vi "String Join.vi"(2 "separator (\\t)":string, 3 "string array":string[](array[string])) -> (0 "joined string":string)   [LabVIEW 2019]
doc: "<b>Description</b> Joins a string array with the specified separator.\n\n<b>Inputs</b>\n<b>separator</b>: \n<b>string array</b>: \n\n<b>Outputs</b>\n<b>joined string</b>: \n\nBSD 3-Clause License\n\nCopyright (c) 2021, TauTerra, LLC\nAll rights reserved.\n\nRedistribution and use in source and binary forms, with or without\nmodification, are permitted provided that the following conditions are met:\n\n1. Redistributions of source code must retain the above copyright notice, this\n list of conditions and the following disclaimer.\n\n2. Redistributions in binary form must reproduce the above copyright notice,\n this list of conditions and the following disclaimer in the documentation\n and/or other materials provided with the distribution.\n\n3. Neither the name of the copyright holder nor the names of its\n contributors may be used to endorse or promote products derived from\n this software without specific prior written permission.\n\nTHIS SOFTWARE IS PROVIDED BY THE COPYRIGHT HOLDERS AND CONTRIBUTORS \"AS IS\"\nAND ANY EXPRESS OR IMPLIED WARRANTIES, INCLUDING, BUT NOT LIMITED TO, THE\nIMPLIED WARRANTIES OF MERCHANTABILITY AND FITNESS FOR A PARTICULAR PURPOSE ARE\nDISCLAIMED. IN NO EVENT SHALL THE COPYRIGHT HOLDER OR CONTRIBUTORS BE LIABLE\nFOR ANY DIRECT, INDIRECT, INCIDENTAL, SPECIAL, EXEMPLARY, OR CONSEQUENTIAL\nDAMAGES (INCLUDING, BUT NOT LIMITED TO, PROCUREMENT OF SUBSTITUTE GOODS OR\nSERVICES; LOSS OF USE, DATA, OR PROFITS; OR BUSINESS INTERRUPTION) HOWEVER\nCAUSED AND ON ANY THEORY OF LIABILITY, WHETHER IN CONTRACT, STRICT LIABILITY,\nOR TORT (INCLUDING NEGLIGENCE OR OTHERWISE) ARISING IN ANY WAY OUT OF THE USE\nOF THIS SOFTWARE, EVEN IF ADVISED OF THE POSSIBILITY OF SUCH DAMAGE."
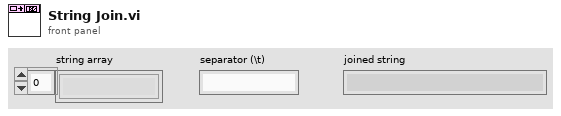
[diagram p1: front panel]
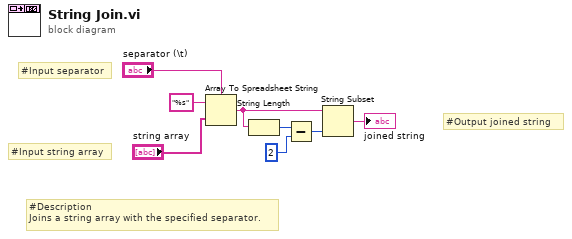
[diagram p0: block diagram]
diagram:
  # "#Output joined string"
  # "#Input separator"
  # "#Input string array"
  # "#Description\nJoins a string array with the specified separator."
  n1 = Array To Spreadsheet String(delimiter (Tab)="separator (\\t)", array="string array", 3:"%s" ("format string")) -> (spreadsheet string=w4:string)
  n2 = String Length(string=w4) -> (length=w3:i32)
  n3 = Subtract(x=w3, y=2 ("x")) -> (x-y=w2:i32)
  n4 = String Subset(string=w4, length (rest)=w2) -> (substring=→"joined string":string)  [unwired: 1 in]
